vi "RisingEdge.vi"(10 "Signal In":bool) -> (2 "Rising Edge":bool)   [LabVIEW 2016, in "kevLib2010.lvlib"]
uses:
  kevLib2010.lvlib
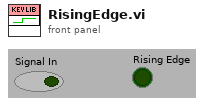
[diagram p1: front panel]
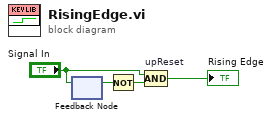
[diagram p0: block diagram]
diagram:
  n1 = feedback-in #1("Signal In") -> ()
  n2 = feedback #1() -> (w3:bool)  [unwired: 1 out]
  n3 = Not(x=w3) -> (.not. x?=w2:bool)
  n4 = Compound Arithmetic op=AND "upReset"("Signal In", w2) -> (→"Rising Edge":bool)
